vi "Untitled 5 (SubVI).vi"(11 "Path":path) -> (3 "Session Generator Output":string)   [LabVIEW 2015]
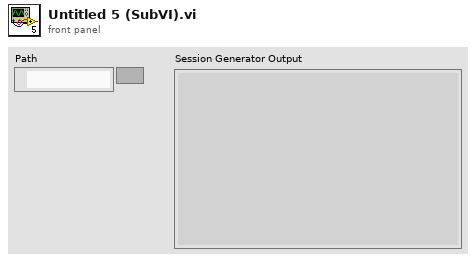
[diagram p1: front panel]
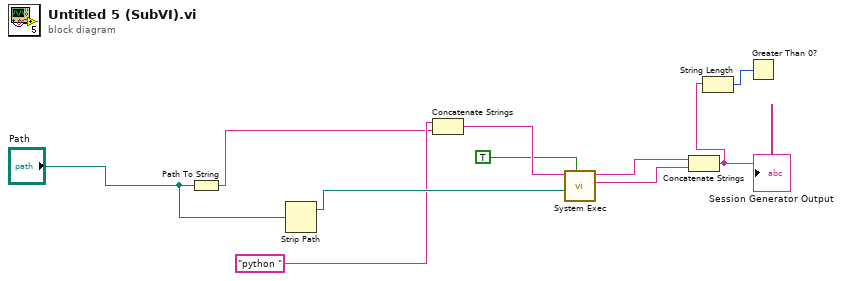
[diagram p0: block diagram]
diagram:
  w3 = TRUE
  n1 = Path To String(path="Path") -> (string=w4:string)
  n2 = Strip Path(path="Path") -> (stripped path=w10:path)  [unwired: 1 out]
  n3 = Concatenate Strings("python ", w4) -> (w5:string)
  n4 = call <vilib>:"System Exec.vi"("run minimized? (F)"=w3, "wait until completion? (T)"=w3, "working directory"=w10, "command line"=w5) -> ("standard error"=w7:string, "standard output"=w6:string)  [unwired: 4 in, 2 out]
  n5 = Concatenate Strings(w6, w7) -> (w2:string)
  "Session Generator Output" <- w2
  n6 = String Length(string=w2) -> (length=w1:i32)
  n7 = Greater Than 0?(x=w1) -> ()  [unwired: 1 out]
